vi "Query List Run State.vi"(8 "error in":errorcluster, 11 "VISA resource name":refnum<visa-resource-name>) -> (0 "error out":errorcluster, 1 "Value":string, 3 "VISA resource name out":refnum<visa-resource-name>)   [LabVIEW 2020, in "IT-M7700.lvlib"]
doc: "This command is used to query the running status of the List."
uses:
  <instrlib>/IT-M7700/IT-M7700.lvlib
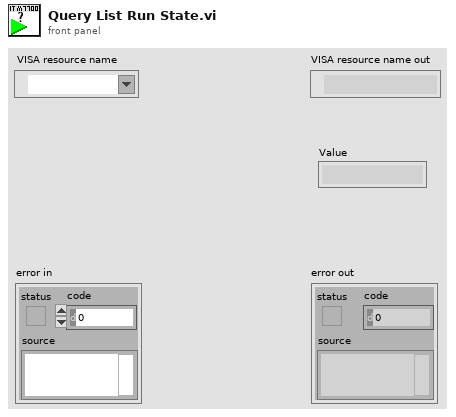
[diagram p1: front panel]
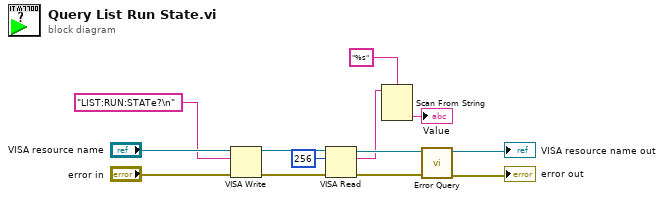
[diagram p0: block diagram]
diagram:
  n1 = VISA Write(VISA resource name="VISA resource name", write buffer="LIST:RUN:STATe?\n", error in (no error)="error in") -> (VISA resource name out=w8:refnum<visa-resource-name>, error out=w7:errorcluster)  [unwired: 1 out]
  n2 = VISA Read(VISA resource name=w8, byte count=u32 256 ("字节总数"), error in (no error)=w7) -> (VISA resource name out=w5:refnum<visa-resource-name>, read buffer=w3:string, error out=w6:errorcluster)  [unwired: 1 out]
  n3 = Scan From String(format string="%s" ("格式字符串"), input string=w3) -> (output 1=→"Value":string)  [unwired: 3 in, 3 out]
  n4 = call <instrlib>:"Error Query.vi"("error in"=w6, "VISA resource name"=w5) -> ("error out"=→"error out":errorcluster, "VISA resource name out"=→"VISA resource name out":refnum<visa-resource-name>)  [unwired: 6 in, 2 out]
